vi "Vision Calculations.vi"(0 "Image In":T2, 3 "error in":errorcluster) -> (5 "Vision Data":T1)   [LabVIEW 2013]
uses:
  <vilib>/vision/Image Controls.llb/IMAQ Image.ctl
  typedefs/vision data.ctl
  <vilib>/vision/NI_Vision_Development_Module.lvlib
panel:
  out "Aspect\nScore":dbl
  out "Rect Score":dbl
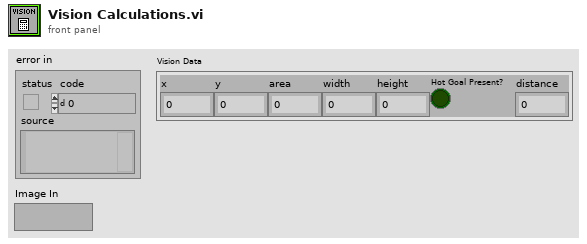
[diagram p1: front panel]
types:
  T1 = typedef "vision data.ctl" = cluster{"x":dbl, "y":dbl, "area":dbl, "width":dbl, "height":dbl, "Hot Goal Present?":bool, "distance":dbl}
  T2 = typedef "IMAQ Image.ctl" = refnum<image>
  T3 = typedef "Particle Parameters" = i32
  T4 = cluster{"Area":dbl, "Number of Holes":dbl, "Bounding Rect":cluster{"Left":dbl, "Top":dbl, "Right":dbl, "Bottom":dbl}, "Center of Mass":cluster{"X":dbl, "Y":dbl}, "Orientation":dbl, "Dimensions":cluster{"Width":dbl, "Height":dbl}}[]
  T5 = cluster{"Horizontal":bool, "Aspect Score":dbl, "Rect Score":dbl, "Rectangle":cluster{"Left":dbl, "Top":dbl, "Right":dbl, "Bottom":dbl}, "Equiv H":dbl, "Equiv V":dbl}
  T6 = cluster{"Area":dbl, "Number of Holes":dbl, "Bounding Rect":cluster{"Left":dbl, "Top":dbl, "Right":dbl, "Bottom":dbl}, "Center of Mass":cluster{"X":dbl, "Y":dbl}, "Orientation":dbl, "Dimensions":cluster{"Width":dbl, "Height":dbl}}
  T7 = cluster{"Left":dbl, "Top":dbl, "Right":dbl, "Bottom":dbl}
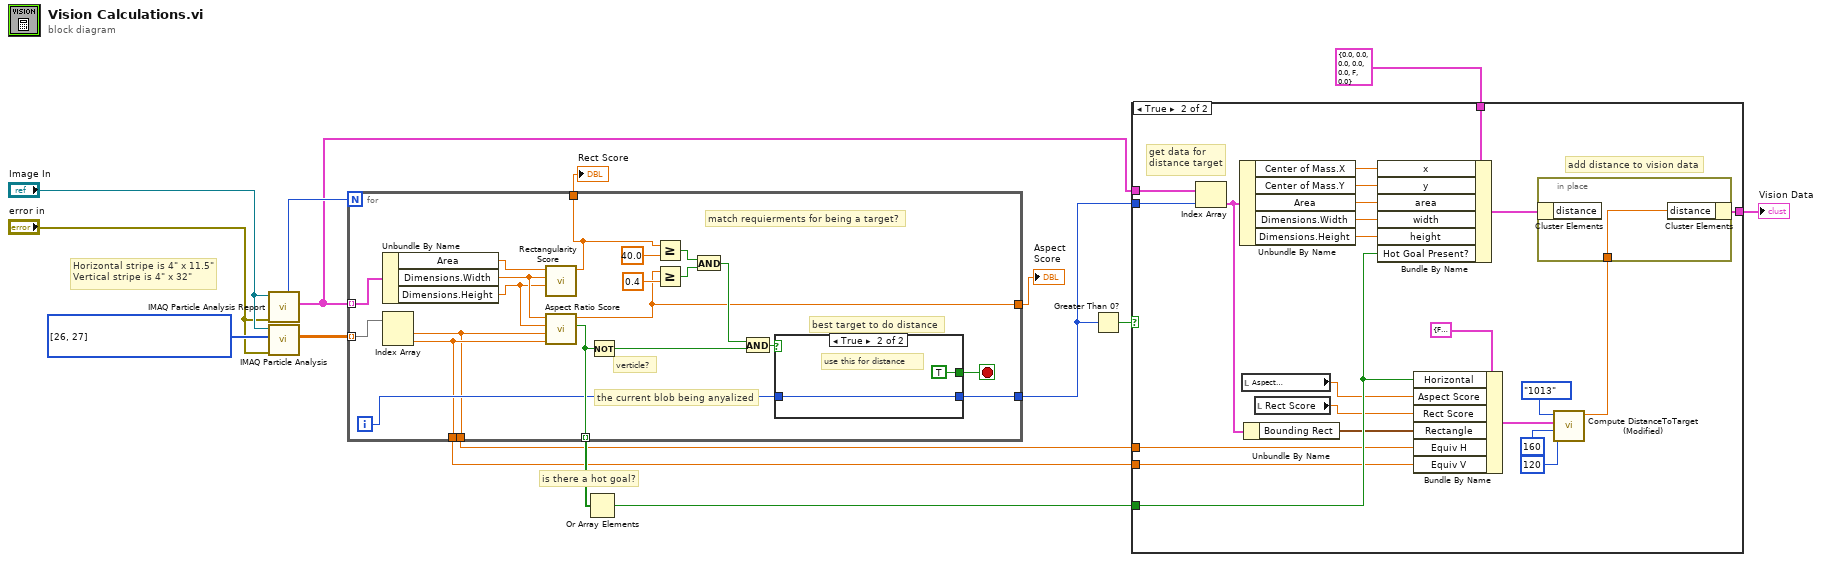
[diagram p0: block diagram]
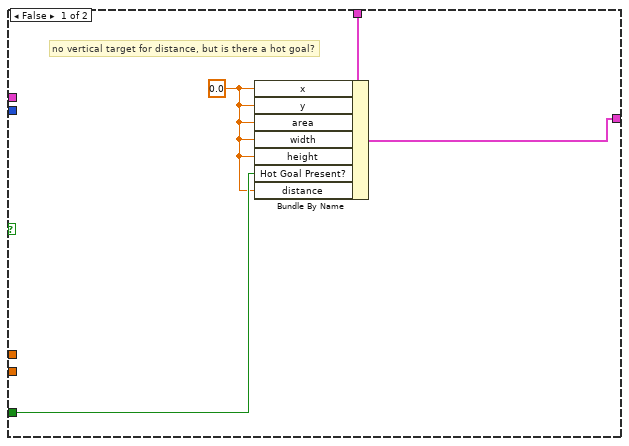
[diagram p2: hidden frame]
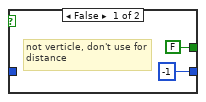
[diagram p3: hidden frame]
diagram:
  w14 = T3[] [26, 27] items=["Center of Mass X", "Center of Mass Y", "First Pixel X", "First Pixel Y", "Bounding Rect Left", "Bounding Rect Top", "Bounding Rect Right", "Bounding Rect Bottom", "Max Feret Diameter Start X", "Max Feret Diameter Start Y", "Max Feret Diameter End X", "Max Feret Diameter End Y", "Max Horiz. Segment Length Left", "Max Horiz. Segment Length Right", "Max Horiz. Segment Length Row", "-", "Bounding Rect Width", "Bounding Rect Height", "Bounding Rect Diagonal", "Perimeter", "Convex Hull Perimeter", "Holes' Perimeter", "Max Feret Diameter", "Equivalent Ellipse Major Axis", "Equivalent Ellipse Minor Axis", "Equivalent Ellipse Minor Axis (Feret)", "Equivalent Rect Long Side", "Equivalent Rect Short Side", "Equivalent Rect Diagonal", "Equivalent Rect Short Side (Feret)", "Average Horiz. Segment Length", "Average Vert. Segment Length", "Hydraulic Radius", "Waddel Disk Diameter", "-", "Area", "Holes' Area", "Particle & Holes' Area", "Convex Hull Area", "Image Area", "-", "Number of Holes", "Number of Horiz. Segments", "Number of Vert. Segments", "-", "Orientation", "Max Feret Diameter Orientation", "-", "% Area/Image Area", "% Area/(Particle & Holes' Area)", "Ratio of Equivalent Ellipse Axes", "Ratio of Equivalent Rect Sides", "-", "Elongation Factor", "Compactness Factor", "Heywood Circularity Factor", "Type Factor", "-", "Sum X", "Sum Y", "Sum XX", "Sum XY", "Sum YY", "Sum XXX", "Sum XXY", "Sum XYY", "Sum YYY", "-", "Moment of Inertia XX", "Moment of Inertia XY", "Moment of Inertia YY", "Moment of Inertia XXX", "Moment of Inertia XXY", "Moment of Inertia XYY", "Moment of Inertia YYY", "Norm. Moment of Inertia XX", "Norm. Moment of Inertia XY", "Norm. Moment of Inertia YY", "Norm. Moment of Inertia XXX", "Norm. Moment of Inertia XXY", "Norm. Moment of Inertia XYY", "Norm. Moment of Inertia YYY", "Hu Moment 1", "Hu Moment 2", "Hu Moment 3", "Hu Moment 4", "Hu Moment 5", "Hu Moment 6", "Hu Moment 7"] ("Pixel Measurements")
  # "Horizontal stripe is 4\" x 11.5\"\nVertical stripe is 4\" x 32\""
  # "is there a hot goal?"
  n1 = call "IMAQ Particle Analysis Report"("error in (no error)"="error in", "Image"="Image In") -> ("Particle Reports (Pixels)"=w10:T4, "Number of Particles"=w16:i32)  [unwired: 4 in, 4 out]
  n2 = call "IMAQ Particle Analysis"("error in (no error)"="error in", "Pixel Measurements"=w14, "Image"="Image In") -> ("Particle Measurements (Pixels)"=w13:dbl[][])  [unwired: 3 in, 5 out]
  n3 = for {
    N: w16 -> [_]
    tunnel: w10 -> [w36] mode=indexing
    tunnel: w13 -> [w35] mode=indexing
    tunnel: [w31] -> w11 mode=indexing
    tunnel: [w23] -> w3
    tunnel: [w20] -> w8
    tunnel: [w19] -> w7
    tunnel: [w18] -> w5
    tunnel: [w17] -> w6
    i -> [w22]
    stop <- w30 stop-if-true
    # "the current blob being anyalized"
    # "match requierments for being a target?"
    # "best target to do distance"
    # "verticle?"
    n4 = Unbundle By Name(w36) -> ("Area"=w34:dbl, "Dimensions.Width"=w33:dbl, "Dimensions.Height"=w32:dbl)
    n5 = Index Array(array=w35) -> (element #1=w17:dbl, element #2=w18:dbl)  [unwired: 2 in]
    n6 = call "Rectangularity Score.vi"("Height"=w32, "Width"=w33, "Area"=w34) -> ("Score"=w20:dbl)  [unwired: 8 in]
    n7 = call "Aspect Ratio Score.vi"("Equivalent Rect Short"=w18, "Equivalent Rect Long"=w17, "Height"=w32, "Width"=w33) -> ("Horizontal"=w31:bool, "Score"=w19:dbl)  [unwired: 6 in]
    n8 = Not(x=w31) -> (.not. x?=w21:bool)
    n9 = Greater Or Equal?(x=w20, y=40.0) -> (x >= y?=w26:bool)
    n10 = Greater Or Equal?(x=w19, y=0.4) -> (x >= y?=w27:bool)
    n11 = And(x=w26, y=w27) -> (x .and. y?=w25:bool)
    n12 = And(x=w25, y=w21) -> (x .and. y?=w24:bool)
    n13 = case shown="True" w24 {
      tunnel: w22 -> [_ w40]
      tunnel: [-1 w40] -> w23
      tunnel: [FALSE TRUE] -> w30
      frame False {
        # "not verticle, don't use for\ndistance"
      }
      frame True {
        # "use this for distance"
      }
    }
  }
  "Rect Score" <- w8
  "Aspect\nScore" <- w7
  n14 = Or Array Elements(Boolean array=w11) -> (logical OR=w9:bool)
  n15 = Greater Than 0?(x=w3) -> (x > 0?=w2:bool)
  n16 = case shown="True" w2 {
    tunnel: w10 -> [_ w67]
    tunnel: w9 -> [w42 w59]
    tunnel: w6 -> [_ w54]
    tunnel: w5 -> [_ w53]
    tunnel: [w43 w48] -> w4
    tunnel: w3 -> [_ w46]
    tunnel: T1 {"x"=0.0, "y"=0.0, "area"=0.0, "width"=0.0, "height"=0.0, "Hot Goal Present?"=FALSE, "distance"=0.0} ("Data") -> [w44 w45]
    frame False {
      w41 = 0.0
      # "no vertical target for distance, but is there a hot goal?"
      n17 = Bundle By Name(cluster=w44, "x"=w41, "y"=w41, "area"=w41, "width"=w41, "height"=w41, "Hot Goal Present?"=w42, "distance"=w41) -> (w43:T1)
    }
    frame True {
      # "add distance to vision data"
      # "get data for \ndistance target"
      n18 = Index Array(array=w67, index=w46) -> (element=w58:T6)
      n19 = Unbundle By Name(w58) -> ("Center of Mass.X"=w66:dbl, "Center of Mass.Y"=w65:dbl, "Area"=w64:dbl, "Dimensions.Width"=w63:dbl, "Dimensions.Height"=w62:dbl)
      n20 = local read "Aspect\nScore"() -> (w55:dbl)
      n21 = Unbundle By Name(w58) -> ("Bounding Rect"=w57:T7)
      n22 = local read "Rect Score"() -> (w56:dbl)
      n23 = Bundle By Name(cluster=w45, "x"=w66, "y"=w65, "area"=w64, "width"=w63, "height"=w62, "Hot Goal Present?"=w59) -> (w49:T1)
      n24 = Bundle By Name(cluster=T5 {"Horizontal"=FALSE, "Aspect Score"=0.0, "Rect Score"=0.0, "Rectangle"={"Left"=0.0, "Top"=0.0, "Right"=0.0, "Bottom"=0.0}, "Equiv H"=0.0, "Equiv V"=0.0} ("Vertical Strip"), "Horizontal"=w59, "Aspect Score"=w55, "Rect Score"=w56, "Rectangle"=w57, "Equiv H"=w54, "Equiv V"=w53) -> (w60:T5)
      n25 = call "Compute DistanceToTarget (Modified).vi"("Y Image Resolution"=120, "X Image Resolution"=160, "Vertical Strip"=w60, "Camera Type"=enum16{"206", "1011", "1013"}."1013") -> ("Distance to Goal Wall (ft)"=w47:dbl)  [unwired: 5 in, 2 out]
      n26 = in-place {
        in-place-border: w47 -> [w68]
        n27 = in-place-cluster #1(w49) -> ()  [unwired: 1 out]
        n28 = in-place-cluster #1("distance"=w68) -> (w48:T1)
      }
    }
  }
  "Vision Data" <- w4
